vi "Persistent_MakePersistent.vi"(7 "Action":T1=enum."GeneratePattern", 8 "error in (no error)":errorcluster, 10 "DataIn":variant, 11 "ClassRefToActOn":refnum<vi>) -> (0 "error out":errorcluster, 1 "Name":string, 2 "DataOut":variant, 3 "Cancelled":bool)   [LabVIEW 2020]
uses:
  <resource>/Framework/Providers/Open_GDS/ClassProviders/Provider_BaseClassInterface/BaseProvider_SubVIs/BaseProvider_DesignPatternsActions.ctl
  <resource>/Framework/Providers/Open_GDS/ClassProviders/Common/LvClass_class/GDSLvClass_ProviderTypes.ctl
  <vilib>/picture/picture.llb/imagedata.ctl
  <vilib>/Utility/miscctls.llb/LVPositionTypeDef.ctl
panel:
  in  "StartAsPersitent":bool
  in  "_Cancel":bool
  in  "_OK":bool
  # "Persistent"
  # "This option will add an input to the New.vi that can make the objects persistent."
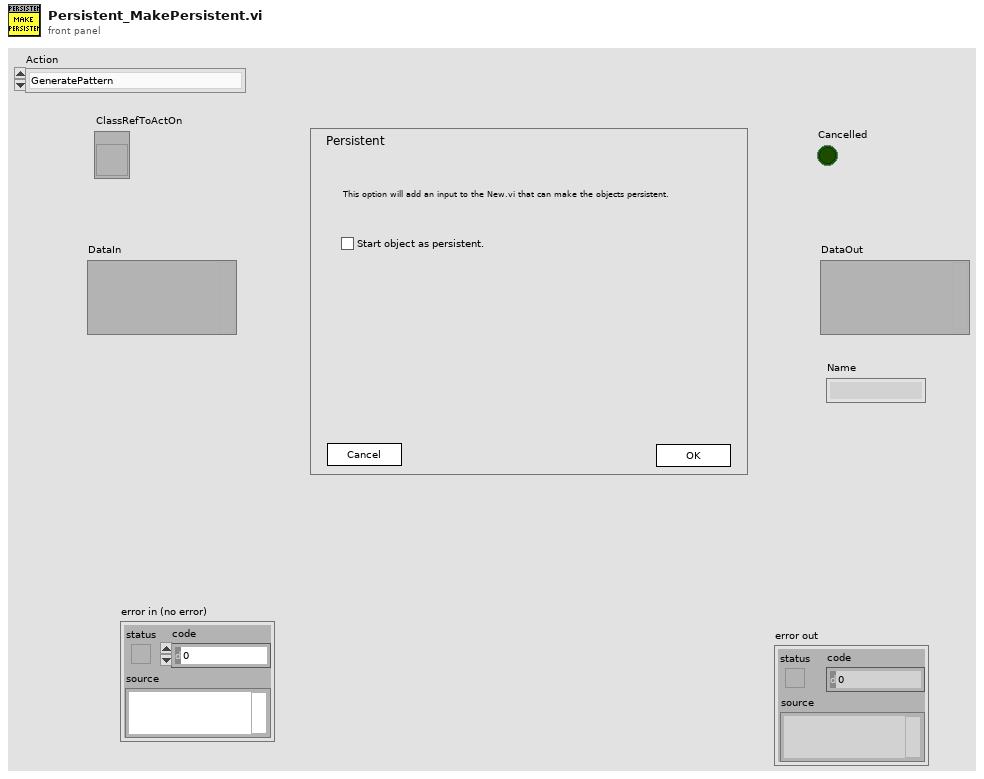
[diagram p1: front panel]
types:
  T1 = typedef "BaseProvider_DesignPatternsActions.ctl" = enum16{"AddPatternDialog", "GeneratePattern", "RemovePattern", "CreatePatternMethod", "UpdatePattern"}
  T2 = typedef "GDSLvClass_ProviderTypes.ctl" = enum16{"UnKnown(LabVOOP)", "Native", "EndevoGOOP3", "OpenG(RootObject)", "OpenG(OpenG_Object)", "EndevoGOOP4", "JKI1"}
  T3 = cluster{"Application":refnum<vi>, "SupportFolder":path, "TemplateName":string, "ClassProvider":T2, "UtilsFolder":path, "UtilsFolderRef":refnum<vi>, "ClassName":string, "Persistent_New.vi":path, "Persistent_CreateReference.vi":path, "NewRef":refnum<vi>, "CreateReferenceRef":refnum<vi>, "ProcessIdRef":refnum<vi>, "TemplateNewRef":refnum<vi>, "StartAsPersitent":bool, "PersistentCPIndex":i32, "FullClassName":string}
  T4 = cluster{"Cancelled":bool, "ClassPath":path, "DataOut":variant, "ClassName":string}
  T5 = enum32{"invalid lock state", "Not Locked", "Locked (No Password)", "Password-protected"}
  T6 = typedef "LVPositionTypeDef.ctl" = cluster{"Left":i32, "Top":i32}
  T7 = typedef "imagedata.ctl" = cluster{"image type":i32, "image depth":i32, "image":u8[], "mask":u8[], "colors":u32[], "Rectangle":cluster{"left":i16, "top":i16, "right":i16, "bottom":i16}}
  T8 = typedef "GDSLvCLass_ClassSettingsType.ctl" = cluster{"ClassProviderName":string, "ClassTemplateUsed":string, "ClassTemplateVersion":string, "ClassDescription":string, "PlugIns":T9[], "ConnectorPanePattern":string}
  T9 = typedef "GDSLvClass_PlugIn.ctl" = cluster{"Type":T10, "ID":string, "Version":string, "Path":path, "Name":string, "Data":variant}
  T10 = typedef "GDSLvClass_PlugInTypes.ctl" = enum16{"DesignPattern", "MethodTypes"}
  T11 = typedef "GDSLvClass_IconSettingsType.ctl" = cluster{"Frame":u32, "Frame thickness":u8, "Header Background":u32, "Header Text":u32, "ColorPublic":u32, "ColorProtected":u32, "ColorPrivate":u32, "Body Text":u32, "ClassBodyIcon":string}
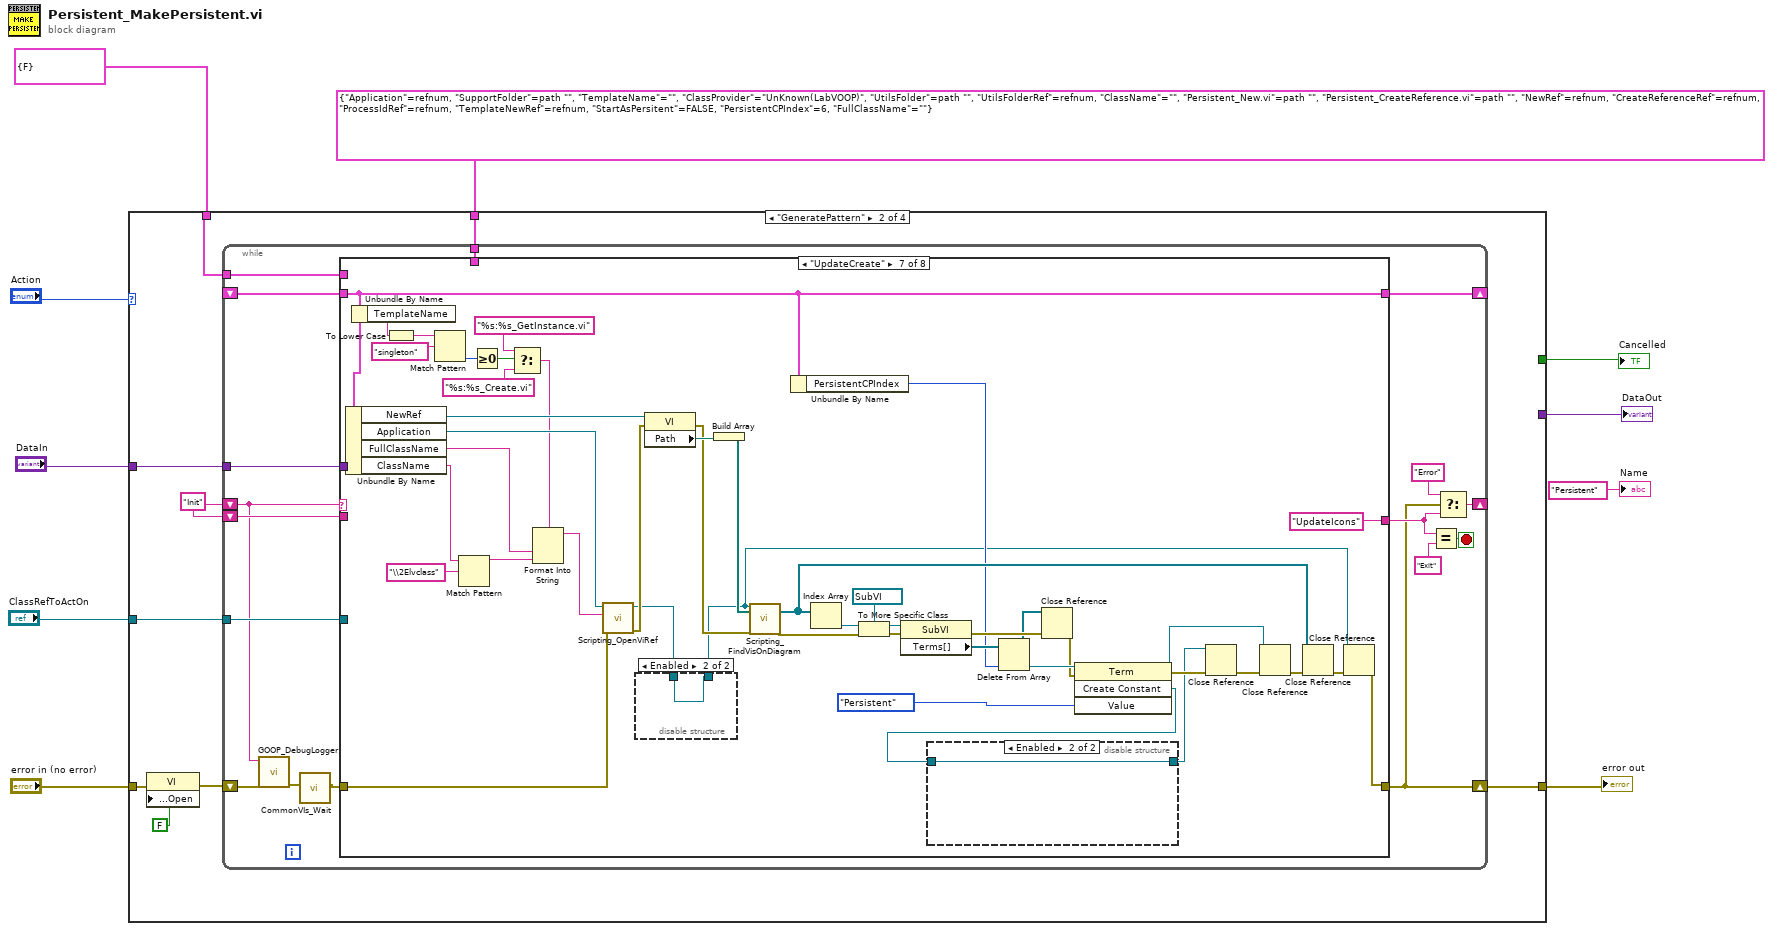
[diagram p0: block diagram]
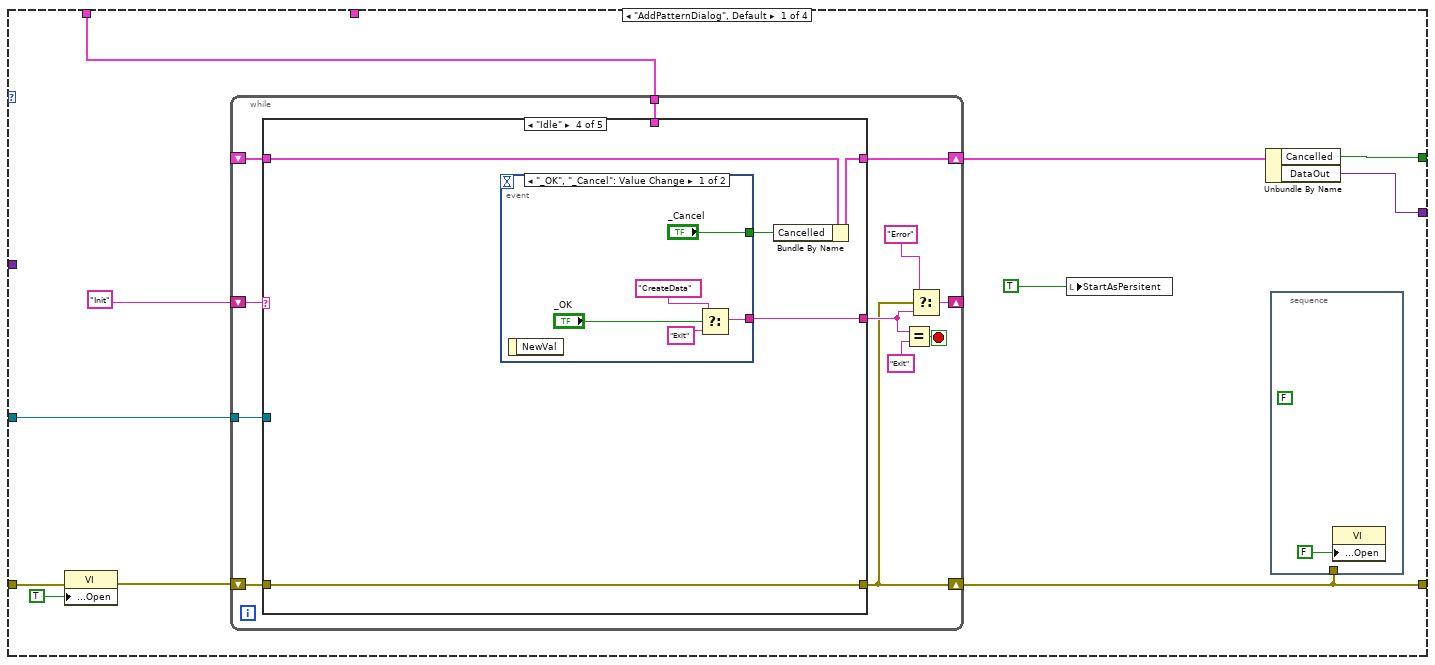
[diagram p2: hidden frame]
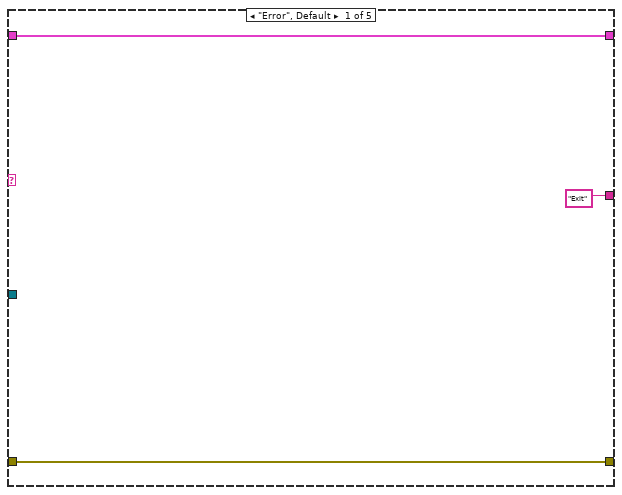
[diagram p3: hidden frame]
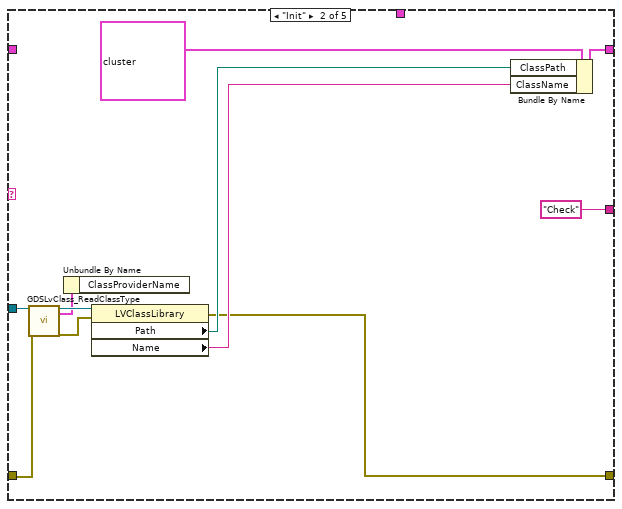
[diagram p4: hidden frame]
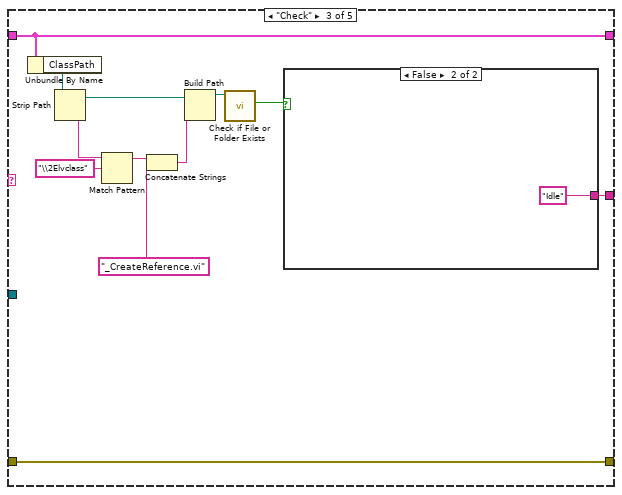
[diagram p5: hidden frame]
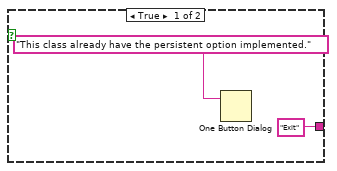
[diagram p6: hidden frame]
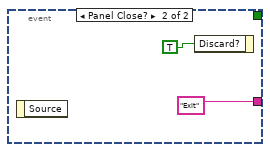
[diagram p7: hidden frame]
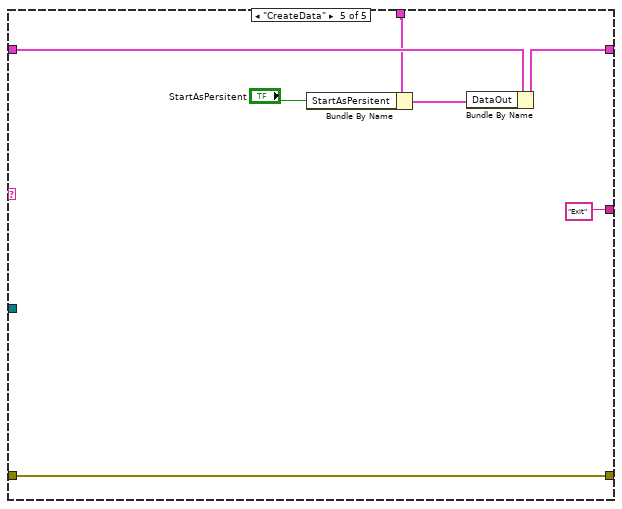
[diagram p8: hidden frame]
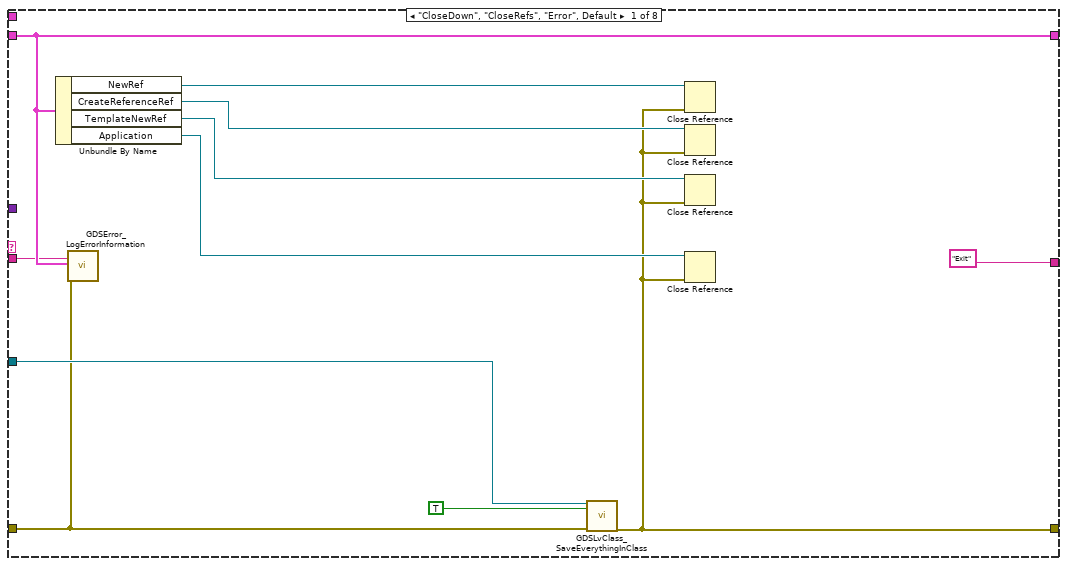
[diagram p9: hidden frame]
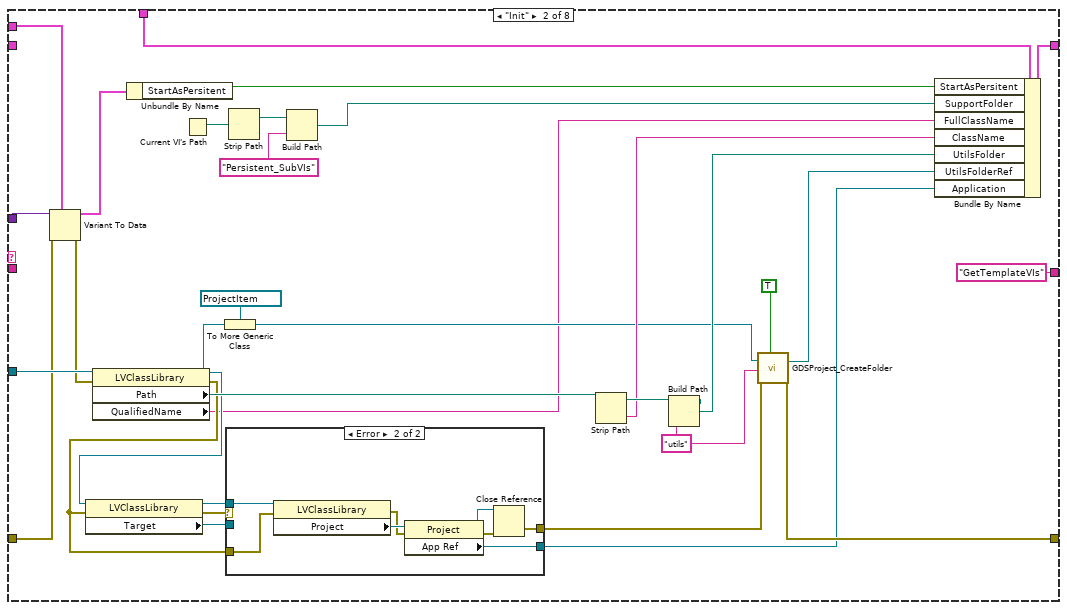
[diagram p10: hidden frame]
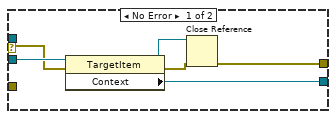
[diagram p11: hidden frame]
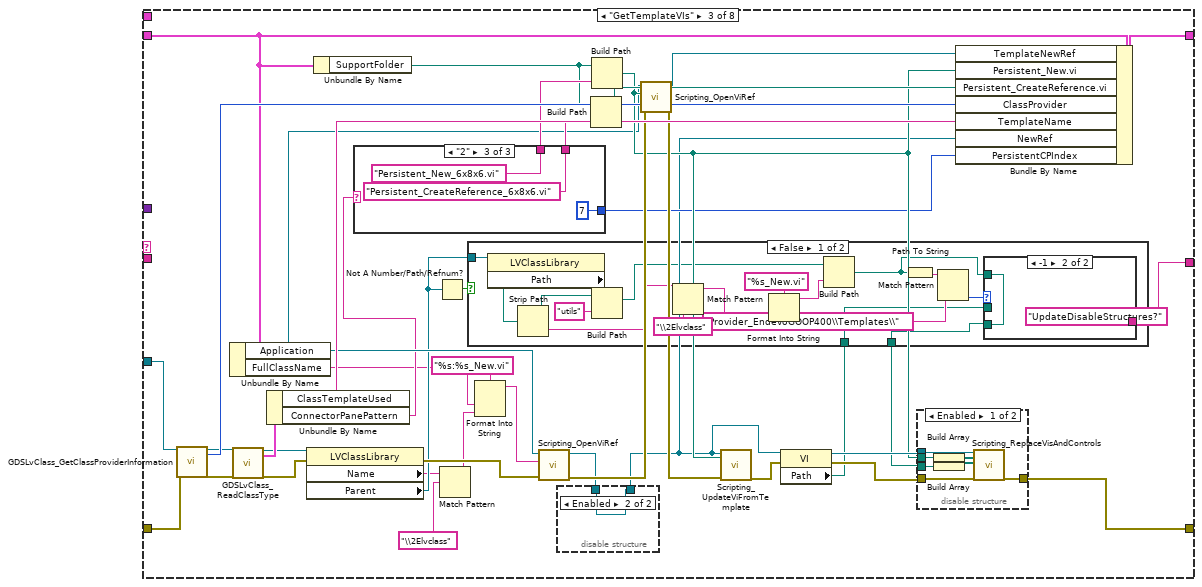
[diagram p12: hidden frame]
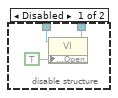
[diagram p13: hidden frame]
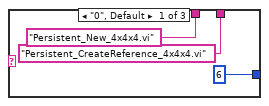
[diagram p14: hidden frame]
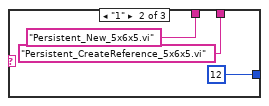
[diagram p15: hidden frame]
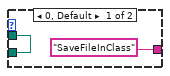
[diagram p16: hidden frame]
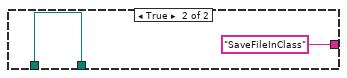
[diagram p17: hidden frame]
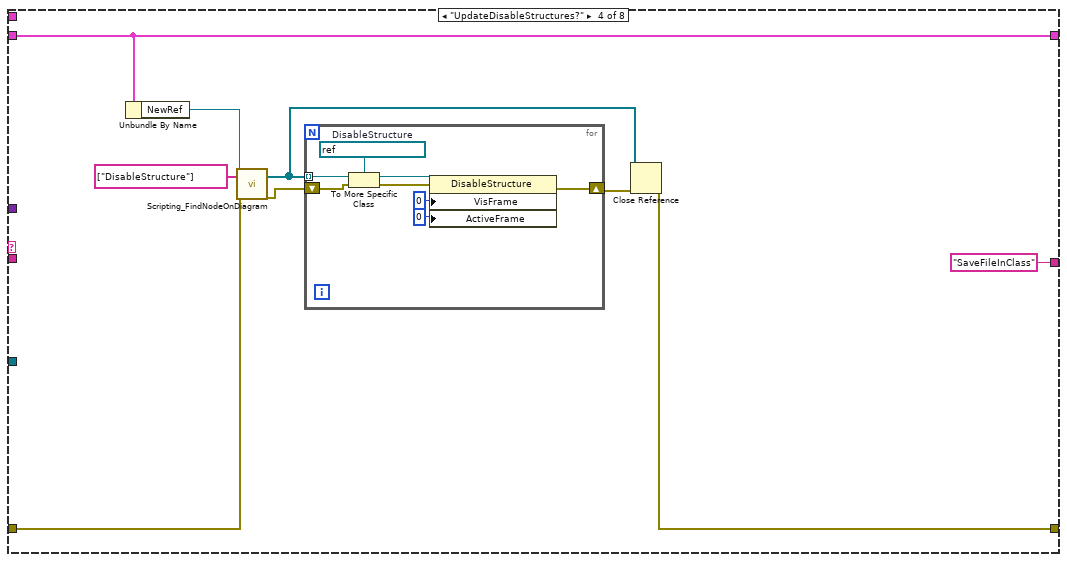
[diagram p19: hidden frame]
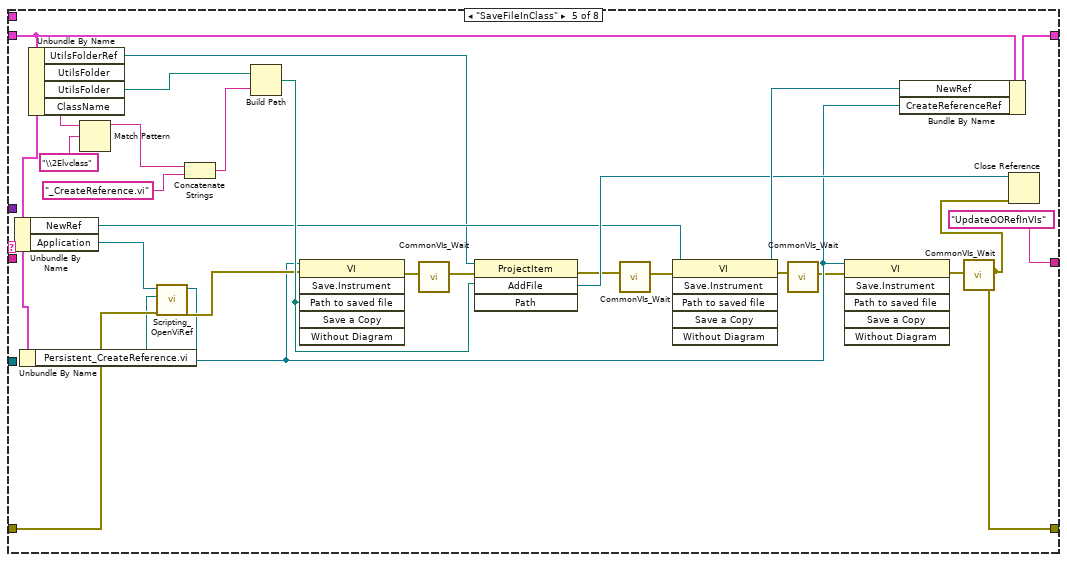
[diagram p20: hidden frame]
diagram:
  n1 = case shown="\"GeneratePattern\"" "Action" {
    tunnel: "error in (no error)" -> [w21 w85 w444 w445]
    tunnel: [w20 w91 w444 w445] -> w8
    tunnel: "ClassRefToActOn" -> [w18 w87 _ _]
    tunnel: [w17 _ _ _] -> w6
    tunnel: [w16 _ _ _] -> w5
    tunnel: cluster{"StartAsPersitent":bool} {"StartAsPersitent"=FALSE} ("output cluster") -> [w15 w89 _ _]
    tunnel: "DataIn" -> [_ w90 _ _]
    tunnel: T3 {"Application"=refnum, "SupportFolder"=path "", "TemplateName"="", "ClassProvider"=enum."UnKnown(LabVOOP)", "UtilsFolder"=path "", "UtilsFolderRef"=refnum, "ClassName"="", "Persistent_New.vi"=path "", "Persistent_CreateReference.vi"=path "", "NewRef"=refnum, "CreateReferenceRef"=refnum, "ProcessIdRef"=refnum, "TemplateNewRef"=refnum, "StartAsPersitent"=FALSE, "PersistentCPIndex"=6, "FullClassName"=""} -> [_ w88 _ _]
    frame "AddPatternDialog", Default {
      n2 = property class="VI"(error in=w21, "Front Panel.Open"=TRUE ("Front Panel Window:Open")) -> (error out=w12:errorcluster)  [unwired: 1 in, 1 out]
      n3 = while {
        shift-right: [w26] -> w20
        shift-left: w12 -> [w33]
        shift-right: [w31] -> _
        shift-left: "Init" -> [w32]
        shift-right: [w25] -> w19
        shift-left: _ -> [w24]
        tunnel: w18 -> [w23]
        tunnel: w15 -> [w22]
        stop <- w30 stop-if-true
        n4 = case shown="\"Idle\"" w32 {
          tunnel: w33 -> [w36 w41 w57 w66 w78]
          tunnel: [w36 w37 w57 w66 w78] -> w26
          tunnel: ["Exit" "Check" w59 w67 "Exit"] -> w27
          tunnel: [w34 w45 w58 w65 w80] -> w25
          tunnel: w24 -> [w34 _ w58 w63 w81]
          tunnel: w23 -> [_ w43 _ _ _]
          tunnel: w22 -> [_ _ _ _ w75]
          frame "Error", Default {
          }
          frame "Init" {
            n5 = call <resource>:"GDSLvClass_ReadClassType.vi"("Class Refnum In"=w43, "error in (no error)"=w41) -> ("Class Refnum Out"=w42:refnum<vi>, "ClassSettings"=w39:T8, "error out"=w40:errorcluster)  [unwired: 15 in]
            n6 = Unbundle By Name(w39) -> ()  [unwired: 1 out]
            n7 = property class="LVClassLibrary"(reference=w42, error in=w40) -> (error out=w37:errorcluster, "Path"=w44:path, "Name"=w38:string)  [unwired: 1 out]
            n8 = Bundle By Name(cluster=T4 {"Cancelled"=FALSE, "ClassPath"=path "", "DataOut"=variant, "ClassName"=""}, "ClassPath"=w44, "ClassName"=w38) -> (w45:T4)
          }
          frame "Check" {
            n9 = Unbundle By Name(w58) -> ("ClassPath"=w56:path)
            n10 = Strip Path(path=w56) -> (stripped path=w50:path, name=w55:string)
            n11 = Match Pattern(string=w55, regular expression="\\2Elvclass") -> (before substring=w53:string)  [unwired: 1 in, 3 out]
            n12 = Concatenate Strings(w53, "_CreateReference.vi" ("element")) -> (w51:string)
            n13 = Build Path(base path=w50, name or relative path=w51) -> (appended path=w49:path)
            n14 = call <vilib>:"Check if File or Folder Exists.vi"("path"=w49) -> ("file or folder exists?"=w48:bool)  [unwired: 8 in, 2 out]
            n15 = case shown="False" w48 {
              tunnel: ["Exit" "Idle"] -> w59
              frame True {
                n16 = One Button Dialog(message="This class already have the persistent option implemented.") -> ()  [unwired: 1 in, 1 out]
              }
              frame False {
              }
            }
          }
          frame "Idle" {
            n17 = event shown="[0] \"_OK\", \"_Cancel\": Value Change" {
              selector: _ -> [_ _]
              dyn-events: _ -> [_ _]
              timeout: _ -> [_ _]
              tunnel: [w71 "Exit"] -> w67
              tunnel: ["_Cancel" _] -> w64
              event "_OK", "_Cancel": Value Change {
                n18 = event-data() -> ()  [unwired: 1 in, 1 out]
                n19 = Select(t="CreateData", s="_OK", f="Exit") -> (s? t:f=w71:string)
              }
              event Panel Close? {
                n20 = event-data() -> ()  [unwired: 1 in, 1 out]
                n21 = event-data("Discard?"=TRUE) -> ()  [unwired: 1 in, 1 out]
              }
            }
            n22 = Bundle By Name(cluster=w63, "Cancelled"=w64) -> (w65:T4)
          }
          frame "CreateData" {
            n23 = Bundle By Name(cluster=w75, "StartAsPersitent"="StartAsPersitent") -> (w76:cluster{"StartAsPersitent":bool})
            n24 = Bundle By Name(cluster=w81, "DataOut"=w76) -> (w80:T4)
          }
        }
        n25 = Equal?(x=w27, y="Exit") -> (x = y?=w30:bool)
        n26 = Select(t="Error", s=w26, f=w27) -> (s? t:f=w31:string)
      }
      n27 = local write "StartAsPersitent"(TRUE ("StartAsPersitent")) -> ()
      n28 = Unbundle By Name(w19) -> ("Cancelled"=w17:bool, "DataOut"=w16:variant)
      n29 = stacked-sequence {
        tunnel: w20 -> [_]
        frame #0 {
          (unwired) FALSE ("Visible")
          n30 = property class="VI"("Front Panel.Open"=FALSE ("Front Panel Window:Open")) -> ()  [unwired: 2 in, 2 out]
        }
      }
    }
    frame "GeneratePattern" {
      w83 = "Init"
      n31 = property class="VI"(error in=w85, "Front Panel.Open"=FALSE ("Front Panel Window:Open")) -> (error out=w84:errorcluster)  [unwired: 1 in, 1 out]
      n32 = while {
        shift-right: [w103] -> w91
        shift-left: w84 -> [w94]
        shift-right: [w108] -> _
        shift-left: w83 -> [w95]
        shift-right: [w102] -> _
        shift-left: _ -> [w101]
        tunnel: w90 -> [w100]
        tunnel: w89 -> [w99]
        tunnel: w88 -> [w98]
        tunnel: w87 -> [w97]
        shift-left: w83 -> [w96]
        stop <- w107 stop-if-true
        n33 = call <resource>:"GOOP_DebugLogger.vi"("error in (no error)"=w94, "State"=w95) -> ("error out"=w93:errorcluster)  [unwired: 7 in, 2 out]
        n34 = call <resource>:"CommonVIs_Wait.vi"("error in"=w93) -> ("error out"=w92:errorcluster)  [unwired: 9 in]
        n35 = case shown="\"UpdateCreate\"" w95 {
          tunnel: w92 -> [w109 w132 w204 w253 w285 w315 w342 w399]
          tunnel: [w112 w141 w187 w252 w267 w304 w362 w398] -> w103
          tunnel: ["Exit" "GetTemplateVIs" w173 "SaveFileInClass" "UpdateOORefInVIs" w296 "UpdateIcons" "CloseRefs"] -> w104
          tunnel: [w111 w150 w202 w251 w293 w298 w346 w401] -> w102
          tunnel: w101 -> [w111 _ w193 w251 w290 w298 w346 w401]
          tunnel: w100 -> [_ w133 _ _ _ _ _ _]
          tunnel: w99 -> [_ w130 _ _ _ _ _ _]
          tunnel: w98 -> [_ w149 _ _ _ _ _ _]
          tunnel: w97 -> [w115 w148 w205 _ _ w314 _ w403]
          tunnel: w96 -> [w110 _ _ _ _ _ _ _]
          frame "CloseDown", "CloseRefs", "Error", Default {
            n36 = Unbundle By Name(w111) -> ("NewRef"=w118:refnum<vi>, "CreateReferenceRef"=w117:refnum<vi>, "TemplateNewRef"=w114:refnum<vi>, "Application"=w113:refnum<vi>)
            n37 = call <resource>:"GDSError_LogErrorInformation.vi"("State"=w110, "LocalVariableData"=w111, "error in (no error)"=w109) -> ()  [unwired: 16 in, 1 out]
            n38 = call <resource>:"GDSLvClass_SaveEverythingInClass.vi"("ClassRefIn"=w115, "ForceResaving(False)"=TRUE, "error in"=w109) -> ("error out"=w112:errorcluster)  [unwired: 15 in, 1 out]
            n39 = Close Reference(reference=w118, error in (no error)=w112) -> ()  [unwired: 1 out]
            n40 = Close Reference(reference=w117, error in (no error)=w112) -> ()  [unwired: 1 out]
            n41 = Close Reference(reference=w114, error in (no error)=w112) -> ()  [unwired: 1 out]
            n42 = Close Reference(reference=w113, error in (no error)=w112) -> ()  [unwired: 1 out]
          }
          frame "Init" {
            w135 = "utils" ("name or relative path")
            n43 = Variant To Data(error in=w132, type=w130, Variant=w133) -> (data=w129:cluster{"StartAsPersitent":bool}, error out=w131:errorcluster)
            n44 = property class="LVClassLibrary"(reference=w148, error in=w131) -> (reference out=w127:refnum<vi>, error out=w121:errorcluster, "Path"=w143:path, "QualifiedName"=w120:string)
            n45 = property class="LVClassLibrary"(reference=w127, error in=w121) -> (reference out=w122:refnum<vi>, error out=w126:errorcluster, "Target"=w125:refnum<vi>)
            n46 = Unbundle By Name(w129) -> ("StartAsPersitent"=w128:bool)
            n47 = Current VI's Path() -> (path=w146:path)
            n48 = To More Generic Class(target class=refnum<vi> refnum ("AddItem"), reference=w127) -> (generic class reference=w134:refnum<vi>)
            n49 = case shown="Error" w126 {
              selector: w126 -> [w153 _]
              tunnel: w125 -> [w157 _]
              tunnel: [w156 w159] -> w124
              tunnel: [w152 w160] -> w123
              tunnel: w122 -> [_ w165]
              tunnel: w121 -> [_ w164]
              frame No Error {
                n50 = property class="TargetItem"(reference=w157, error in=w153) -> (reference out=w154:refnum<vi>, error out=w155:errorcluster, "Context"=w156:refnum<vi>)
                n51 = Close Reference(reference=w154, error in (no error)=w155) -> (error out=w152:errorcluster)
              }
              frame Error {
                n52 = property class="LVClassLibrary"(reference=w165, error in=w164) -> (error out=w158:errorcluster, "Project"=w163:refnum<vi>)  [unwired: 1 out]
                n53 = property class="Project"(reference=w163, error in=w158) -> (reference out=w161:refnum<vi>, error out=w162:errorcluster, "App Ref"=w159:refnum<vi>)
                n54 = Close Reference(reference=w161, error in (no error)=w162) -> (error out=w160:errorcluster)
              }
            }
            n55 = Strip Path(path=w146) -> (stripped path=w145:path)  [unwired: 1 out]
            n56 = Build Path(base path=w145, name or relative path="Persistent_SubVIs") -> (appended path=w139:path)
            n57 = Strip Path(path=w143) -> (stripped path=w140:path, name=w136:string)
            n58 = Build Path(base path=w140, name or relative path=w135) -> (appended path=w137:path)
            n59 = call <resource>:"GDSProject_CreateFolder.vi"("Project Item To Create Folder Below(Use MyComputer if not wired)"=w134, "FolderName"=w135, "error in (no error)"=w123, "CreateThePhysicalFolderIfPossible(False)"=TRUE) -> ("ItemOut"=w138:refnum<vi>, "error out"=w141:errorcluster)  [unwired: 12 in, 2 out]
            n60 = Bundle By Name(cluster=w149, "StartAsPersitent"=w128, "SupportFolder"=w139, "FullClassName"=w120, "ClassName"=w136, "UtilsFolder"=w137, "UtilsFolderRef"=w138, "Application"=w124) -> (w150:T3)
          }
          frame "GetTemplateVIs" {
            n61 = call <resource>:"GDSLvClass_GetClassProviderInformation.vi"("Class Refnum In"=w205, "error in (no error)"=w204) -> ("Class Refnum Out"=w201:refnum<vi>, "ClassProvider"=w203:T2, "error out"=w200:errorcluster)  [unwired: 15 in]
            n62 = Unbundle By Name(w193) -> ("Application"=w175:refnum<vi>, "FullClassName"=w169:string)
            n63 = call <resource>:"GDSLvClass_ReadClassType.vi"("Class Refnum In"=w201, "error in (no error)"=w200) -> ("Class Refnum Out"=w181:refnum<vi>, "ClassSettings"=w199:T8, "error out"=w180:errorcluster)  [unwired: 15 in]
            n64 = Unbundle By Name(w199) -> ("ClassTemplateUsed"=w198:string, "ConnectorPanePattern"=w172:string)
            n65 = property class="LVClassLibrary"(reference=w181, error in=w180) -> (error out=w179:errorcluster, "Name"=w170:string, "Parent"=w174:refnum<vi>)  [unwired: 1 out]
            n66 = Unbundle By Name(w193) -> ("SupportFolder"=w196:path)
            n67 = case shown="\"2\"" w172 {
              tunnel: ["Persistent_New_4x4x4.vi" ("name or relative path") "Persistent_New_5x6x5.vi" ("name or relative path") "Persistent_New_6x8x6.vi" ("name or relative path")] -> w197
              tunnel: ["Persistent_CreateReference_4x4x4.vi" ("name or relative path") "Persistent_CreateReference_5x6x5.vi" ("name or relative path") "Persistent_CreateReference_6x8x6.vi" ("name or relative path")] -> w195
              tunnel: [6 ("PersistentCPIndex") 12 ("PersistentCPIndex") 7 ("PersistentCPIndex")] -> w171
              frame "0", Default {
              }
              frame "1" {
              }
              frame "2" {
              }
            }
            n68 = Not A Number/Path/Refnum?(number/path/refnum=w174) -> (NaN/Path/Refnum?=w178:bool)
            n69 = Match Pattern(string=w170, regular expression="\\2Elvclass") -> (before substring=w168:string)  [unwired: 1 in, 3 out]
            n70 = Format Into String(format string="%s:%s_New.vi", w169, w168) -> (resulting string=w190:string)  [unwired: 2 in, 1 out]
            n71 = call <resource>:"Scripting_OpenViRef.vi"("error in"=w179, "ViPath/ViName/Viref"=w190, "AppRef"=w175) -> ("error out"=w185:errorcluster, "vi reference"=w167:refnum<vi>)  [unwired: 6 in, 1 out]
            n72 = disable-structure shown="Enabled" {
              disable-tunnel: w167 -> [w207 w209]
              disable-tunnel: [w206 w209] -> w166
              frame Disabled {
                n73 = property class="VI"(reference=w207, "BDWin.Open"=TRUE ("Block Diagram Window:Open")) -> (reference out=w206:refnum<vi>)  [unwired: 1 in, 1 out]
              }
              frame Enabled {
              }
            }
            n74 = Build Path(base path=w196, name or relative path=w195) -> (appended path=w194:path)
            n75 = Build Path(base path=w196, name or relative path=w197) -> (appended path=w183:path)
            n76 = call <resource>:"Scripting_OpenViRef.vi"("error in"=w185, "ViPath/ViName/Viref"=w183, "AppRef"=w175) -> ("error out"=w184:errorcluster, "vi reference"=w182:refnum<vi>)  [unwired: 6 in, 1 out]
            n77 = call <resource>:"Scripting_UpdateViFromTemplate.vi"("ViRef"=w166, "TemplateVI(Path or Ref)"=w183, "error in (no error)"=w184) -> ("error out"=w186:errorcluster)  [unwired: 15 in, 1 out]
            n78 = property class="VI"(reference=w166, error in=w186) -> (reference out=w189:refnum<vi>, error out=w188:errorcluster, "Path"=w177:path)
            n79 = case shown="False" w178 {
              tunnel: [w220 w241] -> w176
              tunnel: w177 -> [w219 w241]
              tunnel: w174 -> [w235 _]
              tunnel: [w225 "SaveFileInClass"] -> w173
              frame False {
                n80 = property class="LVClassLibrary"(reference=w235) -> ("Path"=w232:path)  [unwired: 1 in, 2 out]
                n81 = Strip Path(path=w232) -> (stripped path=w230:path, name=w231:string)
                n82 = Build Path(base path=w230, name or relative path="utils") -> (appended path=w228:path)
                n83 = Match Pattern(string=w231, regular expression="\\2Elvclass") -> (before substring=w226:string)  [unwired: 1 in, 3 out]
                n84 = Format Into String(format string="%s_New.vi", w226) -> (resulting string=w227:string)  [unwired: 2 in, 1 out]
                n85 = Build Path(base path=w228, name or relative path=w227) -> (appended path=w221:path)
                n86 = Path To String(path=w221) -> (string=w224:string)
                n87 = Match Pattern(string=w224, regular expression="Provider_EndevoGOOP400\\Templates\\") -> (offset past match=w222:i32)  [unwired: 1 in, 3 out]
                n88 = case shown="-1" w222 {
                  tunnel: ["SaveFileInClass" "UpdateDisableStructures?"] -> w225
                  tunnel: [w236 w238] -> w220
                  tunnel: w221 -> [_ w238]
                  tunnel: w219 -> [w236 _]
                  frame 0, Default {
                  }
                  frame -1 {
                  }
                }
              }
              frame True {
              }
            }
            n89 = disable-structure shown="Enabled" {
              disable-tunnel: w188 -> [w248 w249]
              disable-tunnel: [w247 w249] -> w187
              disable-tunnel: w189 -> [w246 _]
              disable-tunnel: w176 -> [w243 _]
              disable-tunnel: w183 -> [w242 _]
              frame Enabled {
                n90 = Build Array(w242) -> (w245:path[])
                n91 = Build Array(w243) -> (w244:path[])
                n92 = call <resource>:"Scripting_ReplaceVisAndControls.vi"("ViRef"=w246, "OldVIsAndControls"=w245, "NewVIsAndControls"=w244, "error in (no error)"=w248) -> ("error out"=w247:errorcluster)  [unwired: 15 out]
              }
              frame Disabled {
              }
            }
            n93 = Bundle By Name(cluster=w193, "TemplateNewRef"=w182, "Persistent_New.vi"=w183, "Persistent_CreateReference.vi"=w194, "ClassProvider"=w203, "TemplateName"=w198, "NewRef"=w166, "PersistentCPIndex"=w171) -> (w202:T3)
          }
          frame "UpdateDisableStructures?" {
            n94 = Unbundle By Name(w251) -> ("NewRef"=w250:refnum<vi>)
            n95 = call <resource>:"Scripting_FindNodeOnDiagram.vi"("ViRef(Ignored If Not Wired)"=w250, "NodeTypesToSearchFor"=string[] ["DisableStructure"], "error in (no error)"=w253) -> ("Nodes"=w254:refnum<vi>[], "error out"=w256:errorcluster)  [unwired: 15 in]
            n96 = for {
              tunnel: w254 -> [w266] mode=indexing
              shift-right: [w259] -> w255
              shift-left: w256 -> [w264]
              w265 = refnum<vi> refnum  # DisableStructure
              n97 = To More Specific Class(target class=w265, reference=w266, error in=w264) -> (specific class reference=w261:refnum<vi>, error out=w262:errorcluster)
              n98 = property class="DisableStructure"(reference=w261, error in=w262, "VisFrame"=u32 0 ("Visible Frame"), "ActiveFrame"=i16 0 ("Active Frame")) -> (error out=w259:errorcluster)  [unwired: 1 out]
            }
            n99 = Close Reference(reference=w254, error in (no error)=w255) -> (error out=w252:errorcluster)
          }
          frame "SaveFileInClass" {
            n100 = Unbundle By Name(w290) -> ("NewRef"=w276:refnum<vi>, "Application"=w281:refnum<vi>)
            n101 = Unbundle By Name(w290) -> ("Persistent_CreateReference.vi"=w282:path)
            n102 = Unbundle By Name(w290) -> ("UtilsFolderRef"=w275:refnum<vi>, "UtilsFolder"=w277:path, "ClassName"=w289:string)  [unwired: 1 out]
            n103 = Match Pattern(string=w289, regular expression="\\2Elvclass") -> (before substring=w280:string)  [unwired: 1 in, 3 out]
            n104 = call <resource>:"Scripting_OpenViRef.vi"("error in"=w285, "ViPath/ViName/Viref"=w282, "AppRef"=w281) -> ("error out"=w284:errorcluster, "vi reference"=w283:refnum<vi>)  [unwired: 6 in, 1 out]
            n105 = Concatenate Strings(w280, "_CreateReference.vi" ("name or relative path")) -> (w278:string)
            n106 = Build Path(base path=w277, name or relative path=w278) -> (appended path=w287:path)
            n107 = invoke class="VI" method="Save.Instrument"(reference=w283, error in=w284, "Path to saved file"=w287) -> (error out=w272:errorcluster)  [unwired: 3 in, 5 out]
            n108 = call <resource>:"CommonVIs_Wait.vi"("error in"=w272) -> ("error out"=w271:errorcluster)  [unwired: 9 in]
            n109 = invoke class="ProjectItem" method="AddFile"(reference=w275, error in=w271, "Path"=w287) -> (error out=w274:errorcluster, "AddFile"=w286:refnum<vi>)  [unwired: 1 in, 2 out]
            n110 = call <resource>:"CommonVIs_Wait.vi"("error in"=w274) -> ("error out"=w273:errorcluster)  [unwired: 9 in]
            n111 = invoke class="VI" method="Save.Instrument"(reference=w276, error in=w273) -> (reference out=w292:refnum<vi>, error out=w270:errorcluster)  [unwired: 4 in, 4 out]
            n112 = call <resource>:"CommonVIs_Wait.vi"("error in"=w270) -> ("error out"=w269:errorcluster)  [unwired: 9 in]
            n113 = invoke class="VI" method="Save.Instrument"(reference=w283, error in=w269) -> (error out=w268:errorcluster)  [unwired: 4 in, 5 out]
            n114 = Bundle By Name(cluster=w290, "NewRef"=w292, "CreateReferenceRef"=w283) -> (w293:T3)
            n115 = call <resource>:"CommonVIs_Wait.vi"("error in"=w268) -> ("error out"=w267:errorcluster)  [unwired: 9 in]
            n116 = Close Reference(reference=w286, error in (no error)=w267) -> ()  [unwired: 1 out]
          }
          frame "UpdateOORefInVIs" {
            (unwired) "UpdateNew"
            n117 = Unbundle By Name(w298) -> ("Persistent_New.vi"=w303:path, "NewRef"=w311:refnum<vi>, "CreateReferenceRef"=w300:refnum<vi>)
            n118 = Unbundle By Name(w298) -> ("StartAsPersitent"=w297:bool)
            n119 = property class="LVClassLibrary"(reference=w314) -> ("Path"=w301:path)  [unwired: 1 in, 2 out]
            n120 = Path To String(path=w301) -> (string=w312:string)
            n121 = Build Array(w301, w301) -> (w299:path[])
            n122 = Build Array(w311, w300) -> (w313:refnum<vi>[])
            n123 = for {
              tunnel: w313 -> [w327] mode=indexing
              shift-right: [w330] -> w305
              shift-left: w315 -> [w329]
              tunnel: w312 -> [w328]
              tunnel: w301 -> [w326]
              tunnel: path[] [path "LabVIEWClassControl", path "LabVIEWClassConstant"] ("OldVIsAndControls") -> [w325]
              tunnel: w299 -> [w324]
              n124 = disable-structure shown="Enabled" {
                disable-tunnel: [w334 w338] -> w330
                disable-tunnel: w329 -> [w333 w339]
                disable-tunnel: w328 -> [w332 _]
                disable-tunnel: w327 -> [w331 w336]
                disable-tunnel: w326 -> [_ _]
                disable-tunnel: w325 -> [_ w337]
                disable-tunnel: w324 -> [_ w335]
                frame Disabled {
                  n125 = call <resource>:"Scripting_ReplaceOORef.vi"("ViRef"=w331, "NewLvClassFile(ProjectPath or LvClassPath)"=w332, "error in (no error)"=w333) -> ("error out"=w334:errorcluster)  [unwired: 16 in]
                }
                frame Enabled {
                  n126 = call <resource>:"Scripting_ReplaceVisAndControls.vi"("ViRef"=w336, "OldVIsAndControls"=w337, "NewVIsAndControls"=w335, "error in (no error)"=w339) -> ("error out"=w338:errorcluster)  [unwired: 15 out]
                }
              }
            }
            n127 = invoke class="VI" method="Lock State.Set"(reference=w311, error in=w305, "lockState"=T5."Not Locked" ("Lock State")) -> (reference out=w307:refnum<vi>, error out=w306:errorcluster)  [unwired: 4 in, 5 out]
            n128 = property class="VI"(reference=w307, error in=w306) -> (error out=w309:errorcluster, "Path"=w308:path)  [unwired: 1 out]
            n129 = disable-structure shown="Enabled" {
              disable-tunnel: w309 -> [w322 w323]
              disable-tunnel: [w321 w323] -> w304
              disable-tunnel: w300 -> [w320 _]
              disable-tunnel: w308 -> [w317 _]
              disable-tunnel: w303 -> [w316 _]
              frame Enabled {
                n130 = Build Array(w316) -> (w319:path[])
                n131 = Build Array(w317) -> (w318:path[])
                n132 = call <resource>:"Scripting_ReplaceVisAndControls.vi"("ViRef"=w320, "OldVIsAndControls"=w319, "NewVIsAndControls"=w318, "error in (no error)"=w322) -> ("error out"=w321:errorcluster)  [unwired: 15 out]
              }
              frame Disabled {
              }
            }
            n133 = Select(t="UpdateCreate", s=w297, f="UpdateIcons") -> (s? t:f=w296:string)
          }
          frame "UpdateCreate" {
            n134 = Unbundle By Name(w346) -> ("NewRef"=w380:refnum<vi>, "Application"=w381:refnum<vi>, "FullClassName"=w343:string, "ClassName"=w361:string)
            n135 = Unbundle By Name(w346) -> ("TemplateName"=w354:string)
            n136 = To Lower Case(string=w354) -> (all lower case string=w353:string)
            n137 = Match Pattern(string=w353, regular expression="singleton") -> (offset past match=w351:i32)  [unwired: 1 in, 3 out]
            n138 = Match Pattern(string=w361, regular expression="\\2Elvclass") -> (before substring=w383:string)  [unwired: 1 in, 3 out]
            n139 = Greater Or Equal To 0?(x=w351) -> (x >= 0?=w350:bool)
            n140 = Select(t="%s:%s_GetInstance.vi" ("format string"), s=w350, f="%s:%s_Create.vi" ("format string")) -> (s? t:f=w347:string)
            n141 = Format Into String(format string=w347, w343, w383) -> (resulting string=w382:string)  [unwired: 2 in, 1 out]
            n142 = call <resource>:"Scripting_OpenViRef.vi"("error in"=w342, "ViPath/ViName/Viref"=w382, "AppRef"=w381) -> ("error out"=w376:errorcluster, "vi reference"=w341:refnum<vi>)  [unwired: 6 in, 1 out]
            n143 = disable-structure shown="Enabled" {
              disable-tunnel: w341 -> [w386 w388]
              disable-tunnel: [w385 w388] -> w340
              frame Disabled {
                n144 = property class="VI"(reference=w386, "BDWin.Open"=TRUE ("Block Diagram Window:Open")) -> (reference out=w385:refnum<vi>)  [unwired: 1 in, 1 out]
              }
              frame Enabled {
              }
            }
            n145 = property class="VI"(reference=w380, error in=w376) -> (error out=w377:errorcluster, "Path"=w379:path)  [unwired: 1 out]
            n146 = Build Array(w379) -> (w378:path[])
            n147 = call <resource>:"Scripting_FindVisOnDiagram.vi"("ViRef"=w340, "VIsToSerachFor/ViName"=w378, "error in (no error)"=w377) -> ("VisFound"=w365:refnum<vi>[], "error out"=w374:errorcluster)  [unwired: 15 in]
            n148 = Unbundle By Name(w346) -> ("PersistentCPIndex"=w345:i32)
            n149 = Index Array(array=w365) -> (element=w373:refnum<vi>)  [unwired: 1 in]
            n150 = To More Specific Class(target class=refnum<vi> refnum ("WhileLoop"), reference=w373, error in=w374) -> (specific class reference=w372:refnum<vi>, error out=w371:errorcluster)
            n151 = property class="SubVI"(reference=w372, error in=w371) -> (error out=w369:errorcluster, "Terms[]"=w370:refnum<vi>[])  [unwired: 1 out]
            n152 = Delete From Array(array=w370, index=w345) -> (deleted portion=w358:refnum<vi>, array with subset deleted=w359:refnum<vi>[])  [unwired: 1 in]
            n153 = Close Reference(reference=w359, error in (no error)=w369) -> (error out=w357:errorcluster)
            n154 = invoke class="Term" method="Create Constant"(reference=w358, error in=w357, "Value"=enum16{"Default", "Persistent", "NonPersistent"}."Persistent" ("Persistent/Debugging(Default)")) -> (reference out=w366:refnum<vi>, error out=w368:errorcluster, "Create Constant"=w356:refnum<vi>)  [unwired: 1 in, 1 out]
            n155 = disable-structure shown="Enabled" {
              disable-tunnel: w356 -> [w393 w395]
              disable-tunnel: [w392 w395] -> w355
              frame Disabled {
                n156 = property class="Const"(reference=w393) -> (reference out=w394:refnum<vi>, "Position"=w391:T6)  [unwired: 1 in, 1 out]
                n157 = Add(x=w391, y=T6 {"Left"=0, "Top"=16}) -> (x+y=w390:T6)
                n158 = property class="Const"(reference=w394, "Position"=w390) -> (reference out=w392:refnum<vi>)  [unwired: 1 in, 1 out]
              }
              frame Enabled {
              }
            }
            n159 = Close Reference(reference=w355, error in (no error)=w368) -> (error out=w367:errorcluster)
            n160 = Close Reference(reference=w366, error in (no error)=w367) -> (error out=w363:errorcluster)
            n161 = Close Reference(reference=w365, error in (no error)=w363) -> (error out=w364:errorcluster)
            n162 = Close Reference(reference=w340, error in (no error)=w364) -> (error out=w362:errorcluster)
          }
          frame "UpdateIcons" {
            w420 = u8 32 ("x")
            n163 = Unbundle By Name(w401) -> ("CreateReferenceRef"=w402:refnum<vi>, "NewRef"=w396:refnum<vi>)
            n164 = property class="LVClassLibrary"(reference=w403, error in=w399) -> (reference out=w408:refnum<vi>, error out=w404:errorcluster, "Member Data"=w406:refnum<vi>)
            n165 = call <resource>:"GDSLvIcon_AnalyseViIcon.vi"("ViRef/LvCLassRef/LvLibRef/ViPath/2D_Image"=w406, "error in (no error)"=w404) -> ("HeaderIcon"=w409:u8[][], "error out"=w405:errorcluster)  [unwired: 5 in, 11 out]
            n166 = disable-structure shown="Enabled" {
              disable-tunnel: w402 -> [w427 w429]
              disable-tunnel: [w426 w428] -> w397
              disable-tunnel: w396 -> [w425 _]
              frame Disabled {
                n167 = Build Array(w427, w425) -> (w426:refnum<vi>[])
              }
              frame Enabled {
                n168 = Build Array(w429) -> (w428:refnum<vi>[])
              }
            }
            n169 = Close Reference(reference=w406, error in (no error)=w405) -> (error out=w407:errorcluster)
            n170 = Array Size(array=w409) -> (size(s)=w415:i32[])
            n171 = call <resource>:"GDSLvClass_ReadClassColors.vi"("Library Refnum"=w408, "error in (no error)"=w407) -> ("LvClassIconSettings"=w411:T11, "error out"=w400:errorcluster)  [unwired: 12 in, 4 out]
            n172 = Unbundle By Name(w411) -> ("Frame"=w414:u32, "Body Text"=w413:u32, "Frame thickness"=w410:u8)
            n173 = Unbundle By Name(w411) -> ("ColorProtected"=w412:u32)
            n174 = Index Array(array=w415) -> (element #1=w417:i32)  [unwired: 2 in, 1 out]
            n175 = Multiply(x=w410, y=u8 2) -> (x*y=w418:u8)
            n176 = Add(x=w417, y=w418) -> (x+y=w419:i32)
            n177 = Increment(x=w419) -> (x+1=w421:i32)
            n178 = Subtract(x=w420, y=w421) -> (x-y=w422:i32)
            n179 = Subtract(x=w420, y=w418) -> (x-y=w423:u8)
            n180 = for {
              tunnel: w423 -> [_]
              tunnel: w422 -> [_]
              tunnel: w414 -> [w443]
              tunnel: w413 -> [_]
              tunnel: w412 -> [_]
              tunnel: w410 -> [w442]
              tunnel: w409 -> [w441]
              shift-right: [w434] -> w398
              shift-left: w400 -> [w433]
              tunnel: w397 -> [w430] mode=indexing
              n181 = call <resource>:"GDSLvIcon_AnalyseViIcon.vi"("ViRef/LvCLassRef/LvLibRef/ViPath/2D_Image"=w430, "error in (no error)"=w433) -> ("BodyIcon"=w431:u8[][], "error out"=w432:errorcluster)  [unwired: 5 in, 11 out]
              n182 = call <resource>:"GDSLvIcon_CreateIconPicture.vi"("FrameColor"=w443, "FrameThickness(1)"=w442, "HeaderIconIn"=w441, "BodyIconIn"=w431, "error in (no error)"=w432) -> ("WholeIconOut"=w436:u8[][], "error out"=w439:errorcluster)  [unwired: 9 in, 4 out]
              n183 = Reshape Array(w436, 1024 ("dimension size")) -> (w438:u8[])
              n184 = Bundle By Name(cluster=T7 {"image type"=0, "image depth"=8, "image"=[], "mask"=[], "colors"=[], "Rectangle"={"left"=0, "top"=0, "right"=32, "bottom"=32}} ("image data"), "image"=w438) -> (w440:T7)
              n185 = invoke class="VI" method="VI Icon.Set from Image Data"(reference=w430, error in=w439, "ImageData"=w440) -> (error out=w434:errorcluster)  [unwired: 3 in, 5 out]
            }
          }
        }
        n186 = Equal?(x=w104, y="Exit") -> (x = y?=w107:bool)
        n187 = Select(t="Error", s=w103, f=w104) -> (s? t:f=w108:string)
      }
    }
    frame "RemovePattern" {
    }
    frame "CreatePatternMethod" {
    }
  }
  "error out" <- w8
  "DataOut" <- w5
  "Cancelled" <- w6
  "Name" <- "Persistent" ("Name")
